vi "format string.vi"() -> ()   [LabVIEW 2020]
uses:
  <vilib>/Utility/file.llb/Write Delimited Spreadsheet (string).vi
  <vilib>/Utility/file.llb/Read Delimited Spreadsheet (string).vi
  common/features/CF-common_features.lvlib
  <vilib>/Utility/config.llb/NI_LVConfig.lvlib
panel:
  out "size(s)":i32
  out "deleted portion":string[][](array[string])
  out "length":i32
  out "all rows":string[][](array[string])
  out "string array 3":string[](array[string])
  out "string array 2":string[](array[string])
  out "string array":string[](array[string])
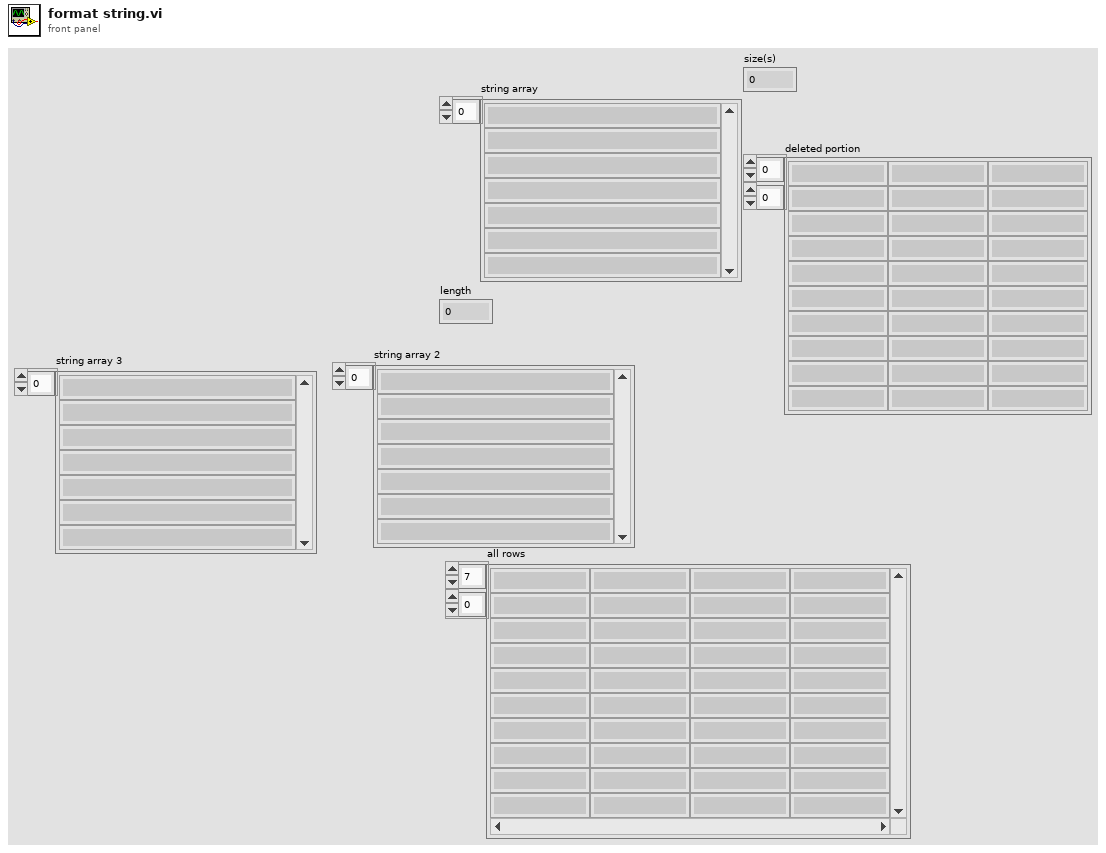
[diagram p1: front panel]
types:
  T1 = enum16{"open", "replace", "create", "open or create", "replace or create", "replace or create with confirmation"}
  T2 = cluster{"software":string, "date":string, "config info":string, "signal name":string, "info":string, "signals":string, "sdsad":string}
  T3 = typedef "NI_LVConfig.lvlib/Config Data RefNum.ctl" = refnum<k1>
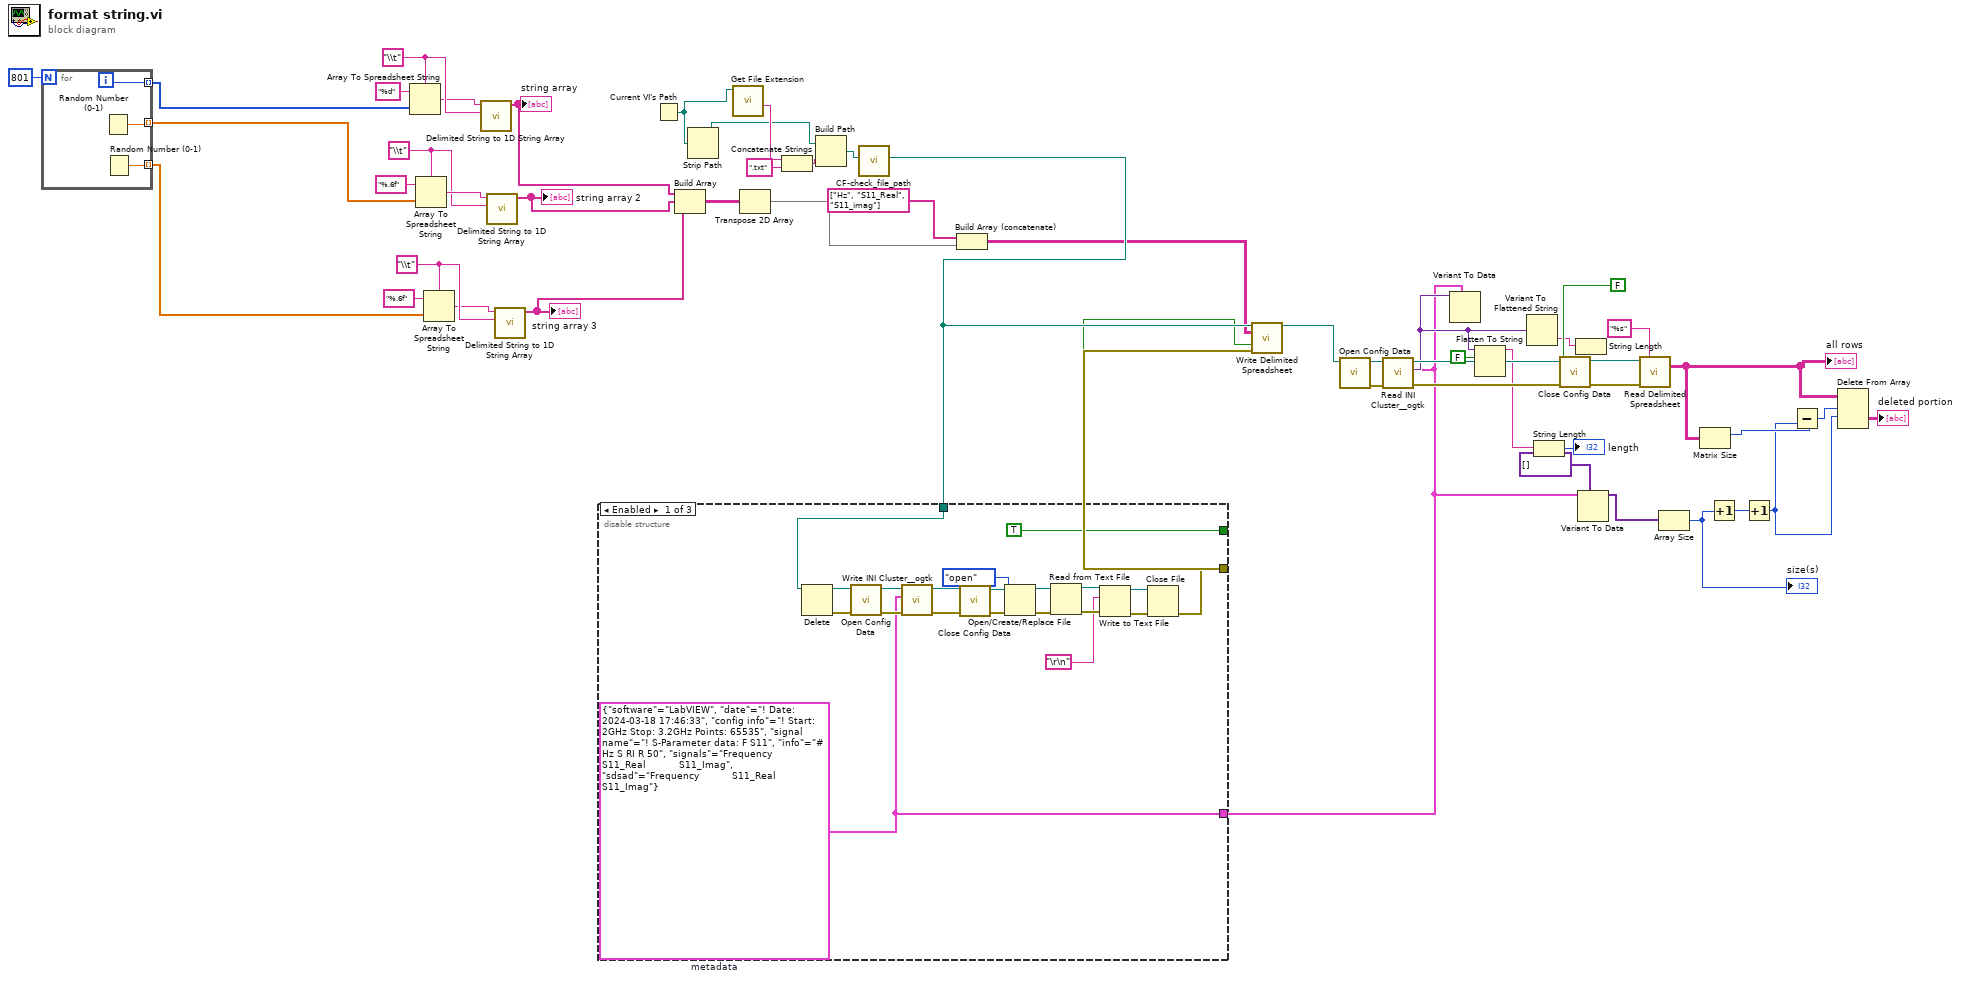
[diagram p0: block diagram]
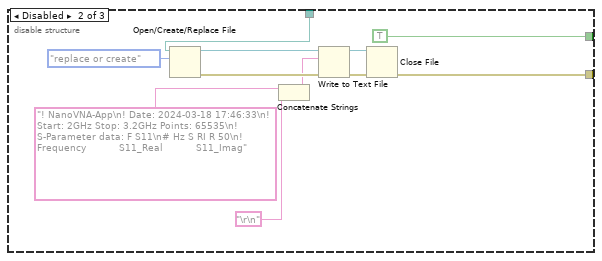
[diagram p2: hidden frame]
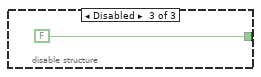
[diagram p3: hidden frame]
diagram:
  w43 = "\\t" ("delimiter (Tab)")
  w47 = "\\t" ("delimiter (Tab)")
  w50 = "\\t" ("delimiter (Tab)")
  n1 = for {
    N: 801 -> [_]
    tunnel: [w56] -> w45 mode=indexing
    tunnel: [w55] -> w41 mode=indexing
    tunnel: [w54] -> w52 mode=indexing
    i -> [w54]
    n2 = Random Number (0-1)() -> (number: 0 to 1=w56:dbl)
    n3 = Random Number (0-1)() -> (number: 0 to 1=w55:dbl)
  }
  n4 = Array To Spreadsheet String(delimiter (Tab)=w50, array=w52, 3:"%d" ("format string")) -> (spreadsheet string=w49:string)
  n5 = Array To Spreadsheet String(delimiter (Tab)=w47, array=w45, 3:"%.6f" ("format string")) -> (spreadsheet string=w48:string)
  n6 = Array To Spreadsheet String(delimiter (Tab)=w43, array=w41, 3:"%.6f" ("format string")) -> (spreadsheet string=w42:string)
  n7 = call <vilib>:"Delimited String to 1D String Array.vi"("delimiter"=w50, "delimited string"=w49) -> ("string array"=w40:string[])  [unwired: 9 in]
  "string array" <- w40
  n8 = call <vilib>:"Delimited String to 1D String Array.vi"("delimiter"=w47, "delimited string"=w48) -> ("string array"=w39:string[])  [unwired: 9 in]
  "string array 2" <- w39
  n9 = call <vilib>:"Delimited String to 1D String Array.vi"("delimiter"=w43, "delimited string"=w42) -> ("string array"=w38:string[])  [unwired: 9 in]
  "string array 3" <- w38
  n10 = Current VI's Path() -> (path=w37:path)
  n11 = Build Array(w40, w39, w38) -> (w31:string[][])
  n12 = Strip Path(path=w37) -> (stripped path=w35:path)  [unwired: 1 out]
  n13 = call <vilib>:"Get File Extension.vi"("file"=w37) -> ("filename without extension"=w36:string)  [unwired: 6 in, 4 out]
  n14 = Transpose 2D Array(2D array=w31) -> (transposed array=w4:string[][])
  n15 = Concatenate Strings(w36, ".txt" ("string")) -> (w34:string)
  n16 = Build Path(base path=w35, name or relative path=w34) -> (appended path=w32:path)
  n17 = call "CF-check_file_path.vi"("File Path"=w32) -> ("File Path out"=w30:path)  [unwired: 10 in]
  n18 = disable-structure shown="Enabled" {
    disable-tunnel: [w64 w83 _] -> w29
    disable-tunnel: w30 -> [w70 w81 _]
    disable-tunnel: [TRUE ("append to file? (new file:F)") TRUE ("append to file? (new file:F)") FALSE ("append to file? (new file:F)")] -> w28
    disable-tunnel: [w57 _ _] -> w8
    frame Enabled {
      w57 = T2 {"software"="LabVIEW", "date"="! Date: 2024-03-18 17:46:33", "config info"="! Start: 2GHz Stop: 3.2GHz Points: 65535", "signal name"="! S-Parameter data: F S11", "info"="# Hz S RI R 50", "signals"="Frequency           S11_Real           S11_Imag", "sdsad"="Frequency           S11_Real           S11_Imag"}  # metadata
      n19 = Delete(path (use dialog)=w70) -> (deleted path=w69:path, error out=w71:errorcluster)  [unwired: 4 in, 1 out]
      n20 = call <vilib>:"Open Config Data.vi"("error in (no error)"=w71, "configuration file path"=w69) -> ("error out"=w72:errorcluster, "refnum"=w73:T3)  [unwired: 7 in, 1 out]
      n21 = call <userlib>:"Write INI Cluster__ogtk.vi"("error in (no error)"=w72, "INI Fomatted Cluster"=w57, "refnum"=w73) -> ("error out"=w75:errorcluster, "dup refnum"=w74:T3)  [unwired: 7 in]
      n22 = call <vilib>:"Close Config Data.vi"("error in (no error)"=w75, "refnum"=w74) -> ("error out"=w65:errorcluster, "file path"=w66:path)  [unwired: 8 in]
      n23 = Open/Create/Replace File(file path (use dialog)=w66, error in=w65, operation (0:open)=T1."open") -> (refnum out=w61:refnum<file>, error out=w62:errorcluster)  [unwired: 3 in, 1 out]
      n24 = Read from Text File(file (use dialog)=w61, error in=w62) -> (refnum out=w60:refnum<file>, error out=w59:errorcluster)  [unwired: 2 in, 2 out]
      n25 = Write to Text File(file (use dialog)=w60, text="\r\n", error in=w59) -> (refnum out=w67:refnum<file>, error out=w68:errorcluster)  [unwired: 1 in, 1 out]
      n26 = Close File(refnum=w67, error in=w68) -> (error out=w64:errorcluster)  [unwired: 1 out]
    }
    frame Disabled {
      n27 = Open/Create/Replace File(file path (use dialog)=w81, operation (0:open)=T1."replace or create") -> (refnum out=w84:refnum<file>, error out=w85:errorcluster)  [unwired: 4 in, 1 out]
      n28 = Concatenate Strings("! NanoVNA-App\n! Date: 2024-03-18 17:46:33\n! Start: 2GHz Stop: 3.2GHz Points: 65535\n! S-Parameter data: F S11\n# Hz S RI R 50\n!     Frequency           S11_Real           S11_Imag" ("text"), "\r\n") -> (w77:string)
      n29 = Write to Text File(file (use dialog)=w84, text=w77, error in=w85) -> (refnum out=w86:refnum<file>, error out=w87:errorcluster)  [unwired: 1 in, 1 out]
      n30 = Close File(refnum=w86, error in=w87) -> (error out=w83:errorcluster)  [unwired: 1 out]
    }
    frame Disabled {
    }
  }
  n31 = Build Array (concatenate)(string[] ["Hz", "S11_Real", "S11_imag"] ("element"), w4) -> (w2:string[][])
  n32 = call-poly <vilib>:"Write Delimited Spreadsheet.vi"("file path (dialog if empty)"=w30, "2D data"=w2, "append to file? (new file:F)"=w28, "error in (no error)"=w29) -> ("new file path (Not A Path if cancelled)"=w23:path)  [unwired: 10 in, 1 out]
  n33 = call <vilib>:"Open Config Data.vi"("configuration file path"=w23) -> ("error out"=w24:errorcluster, "refnum"=w27:T3)  [unwired: 8 in, 1 out]
  n34 = call <userlib>:"Read INI Cluster__ogtk.vi"("error in (no error)"=w24, "INI Fomatted Cluster Type"=w8, "refnum"=w27) -> ("error out"=w25:errorcluster, "INI Fomatted Cluster"=w17:variant, "dup refnum"=w26:T3)  [unwired: 4 in, 2 out]
  n35 = Variant To Data(type=w8, Variant=w17) -> ()  [unwired: 1 in, 2 out]
  n36 = Flatten To String(anything=w17, prepend array or string size? (T)=FALSE) -> (data string=w15:string)  [unwired: 2 in, 2 out]
  n37 = Variant To Flattened String(Variant=w17) -> (data string=w18:string)  [unwired: 1 out]
  n38 = String Length(string=w15) -> (length=→"length":i32)
  n39 = call <vilib>:"Close Config Data.vi"("error in (no error)"=w25, "write file if changed (T)"=FALSE, "refnum"=w26) -> ("error out"=w22:errorcluster, "file path"=w21:path)  [unwired: 7 in]
  n40 = String Length(string=w18) -> ()  [unwired: 1 out]
  n41 = Variant To Data(type=variant[] [], Variant=w8) -> (data=w7:variant[])  [unwired: 1 in, 1 out]
  n42 = call-poly <vilib>:"Read Delimited Spreadsheet.vi"("file path (dialog if empty)"=w21, "format (%s)"="%s" ("format (%.3f)"), "error in (no error)"=w22) -> ("all rows"=w13:string[][])  [unwired: 7 in, 5 out]
  "all rows" <- w13
  n43 = Array Size(array=w7) -> (size(s)=w6:i32)
  "size(s)" <- w6
  n44 = Matrix Size(0:w13) -> (1:w12:i32)  [unwired: 1 out]
  n45 = Increment(x=w6) -> (x+1=w5:i32)
  n46 = Increment(x=w5) -> (x+1=w1:i32)
  n47 = Subtract(x=w12, y=w1) -> (x-y=w11:i32)
  n48 = Delete From Array(array=w13, length=w11, index (row)=w1) -> (deleted portion=→"deleted portion":string[][])  [unwired: 1 in, 1 out]
